vi "View-User Colors.vi"(11 "Material-Scheme.lvclass":refnum<class "Material-Scheme.lvclass">) -> ()   [LabVIEW 2021, in "TSC Material Theme.lvlib" / "Material-Scheme.lvclass"]
doc: "Allow developers to copy the colors from the scheme or save to the <i>User Colors</i> in the LabVIEW Configuration. \n\n<b>Note:</b> Updates to User Colors in the LabVIEW Config File require a restart\n\n<b>Code Developed By:</b>\nTechnology Service Corporation\nwww.tsc.com/atcs\n\nDeveloper:\nDaniel Coons"
uses:
  Material-Scheme.lvclass
  <vilib>/Utility/traverseref.llb/TRef TravTarget.ctl
  Material-Scheme.lvclass/Material-Scheme.ctl
  a595172c-2363-402c-a87e-7fcaa5b8fa44.vi
  <vilib>/Utility/colorconv.llb/Color to RGB.vi
  <vilib>/Comparison/Less/Less Functor/Less Functor.lvclass
  <vilib>/Utility/traverseref.llb/VI Scripting - Traverse.lvlib
panel:
  in  "exit":bool
  in  "stop VI":bool caption="This will FP Open to copy colors.\nUse Get Color tool or right click\nto copy color data."
  in  "restore LabVIEW defaults\nfor User Colors":bool
  in  "update User Colors":bool
  in  "deselect all":bool
  in  "default suggestions":bool
  out "selections":i32 caption="Numeric"
  in  "choices":bool[](array[boolean])
  out "color names":string[](array[string])
  out "Scrim":u32(colorbox)
  out "Shadow":u32(colorbox)
  out "Inverse Primary":u32(colorbox)
  out "Inverse on Surface":u32(colorbox)
  out "Inverse Surface":u32(colorbox)
  out "Outline Variant":u32(colorbox)
  out "Outline":u32(colorbox)
  out "On Surface Var":u32(colorbox)
  out "On Surface":u32(colorbox)
  out "Surf Container Highest":u32(colorbox)
  out "Surf Container High":u32(colorbox)
  out "Surf Container":u32(colorbox)
  out "Surf Container Low":u32(colorbox)
  out "Surf Container Lowest":u32(colorbox)
  out "Surface Bright":u32(colorbox)
  out "Surface":u32(colorbox)
  out "Surface Dim":u32(colorbox)
  out "On Error Container":u32(colorbox)
  out "Error Container":u32(colorbox)
  out "On Error":u32(colorbox)
  out "Error":u32(colorbox)
  out "On Tertiary Fixed Variant":u32(colorbox)
  out "On Tertiary Fixed":u32(colorbox)
  out "Tertiary Fixed Dim":u32(colorbox)
  out "Tertiary Fixed":u32(colorbox)
  out "On Tertiary Container":u32(colorbox)
  out "Tertiary Container":u32(colorbox)
  out "On Tertiary":u32(colorbox)
  out "Tertiary":u32(colorbox)
  out "On Secondary Fixed Variant":u32(colorbox)
  out "On Secondary Fixed":u32(colorbox)
  out "Secondary Fixed Dim":u32(colorbox)
  out "Secondary Fixed":u32(colorbox)
  out "On Secondary Container":u32(colorbox)
  out "Secondary Container":u32(colorbox)
  out "On Secondary":u32(colorbox)
  out "Secondary":u32(colorbox)
  out "On Primary Fixed Variant":u32(colorbox)
  out "On Primary Fixed":u32(colorbox)
  out "Primary Fixed Dim":u32(colorbox)
  out "Primary Fixed":u32(colorbox)
  out "On Primary Container":u32(colorbox)
  out "Primary Container":u32(colorbox)
  out "On Primary":u32(colorbox)
  out "Primary":u32(colorbox)
  out "hex colors":string[](array[string])
  # "developer can select\na maximum of 18 colors"
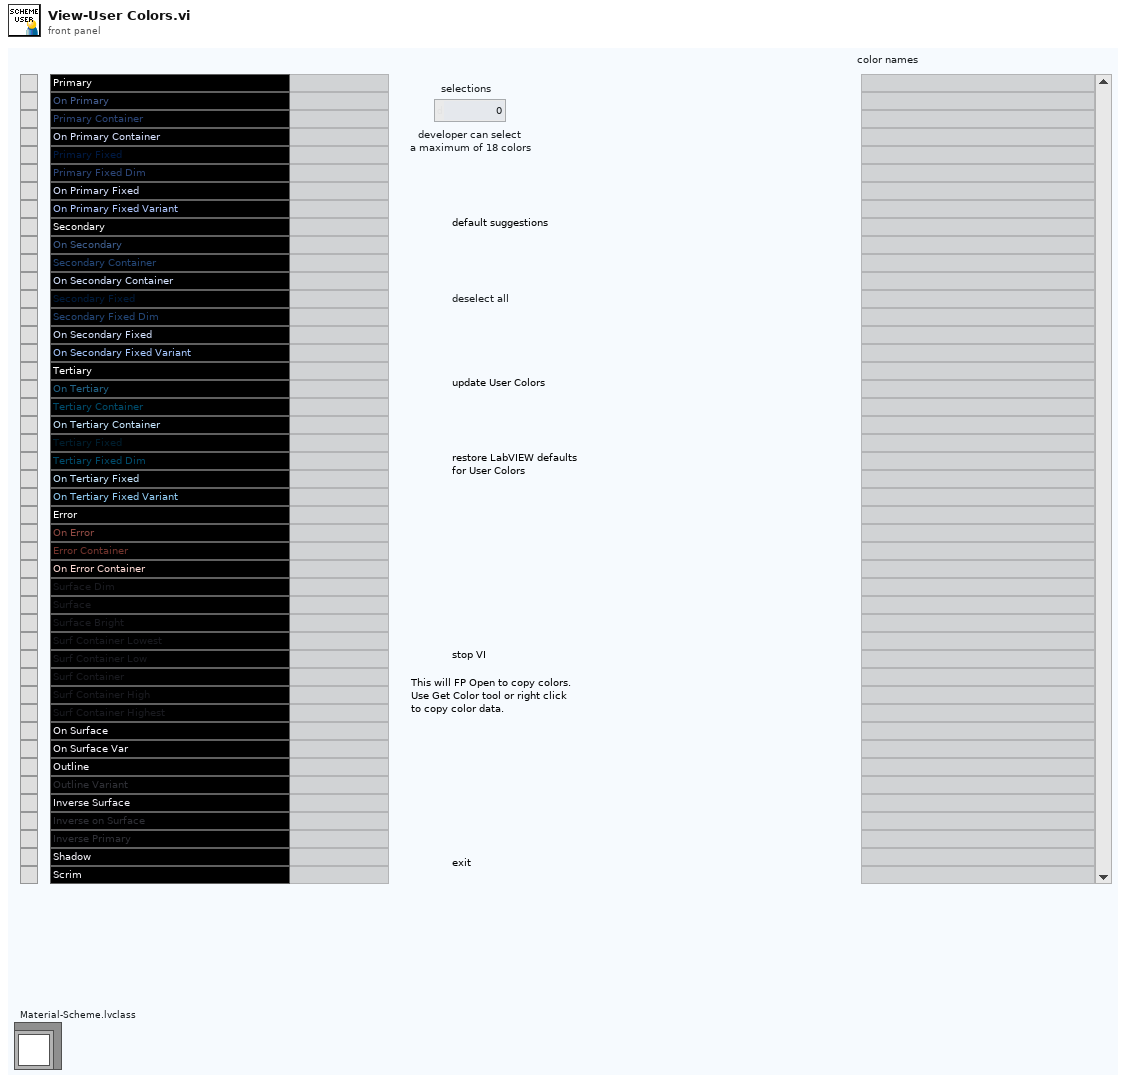
[diagram p1: front panel]
types:
  T1 = typedef "TRef TravTarget.ctl" = enum16{"FP", "BD", "Other"}
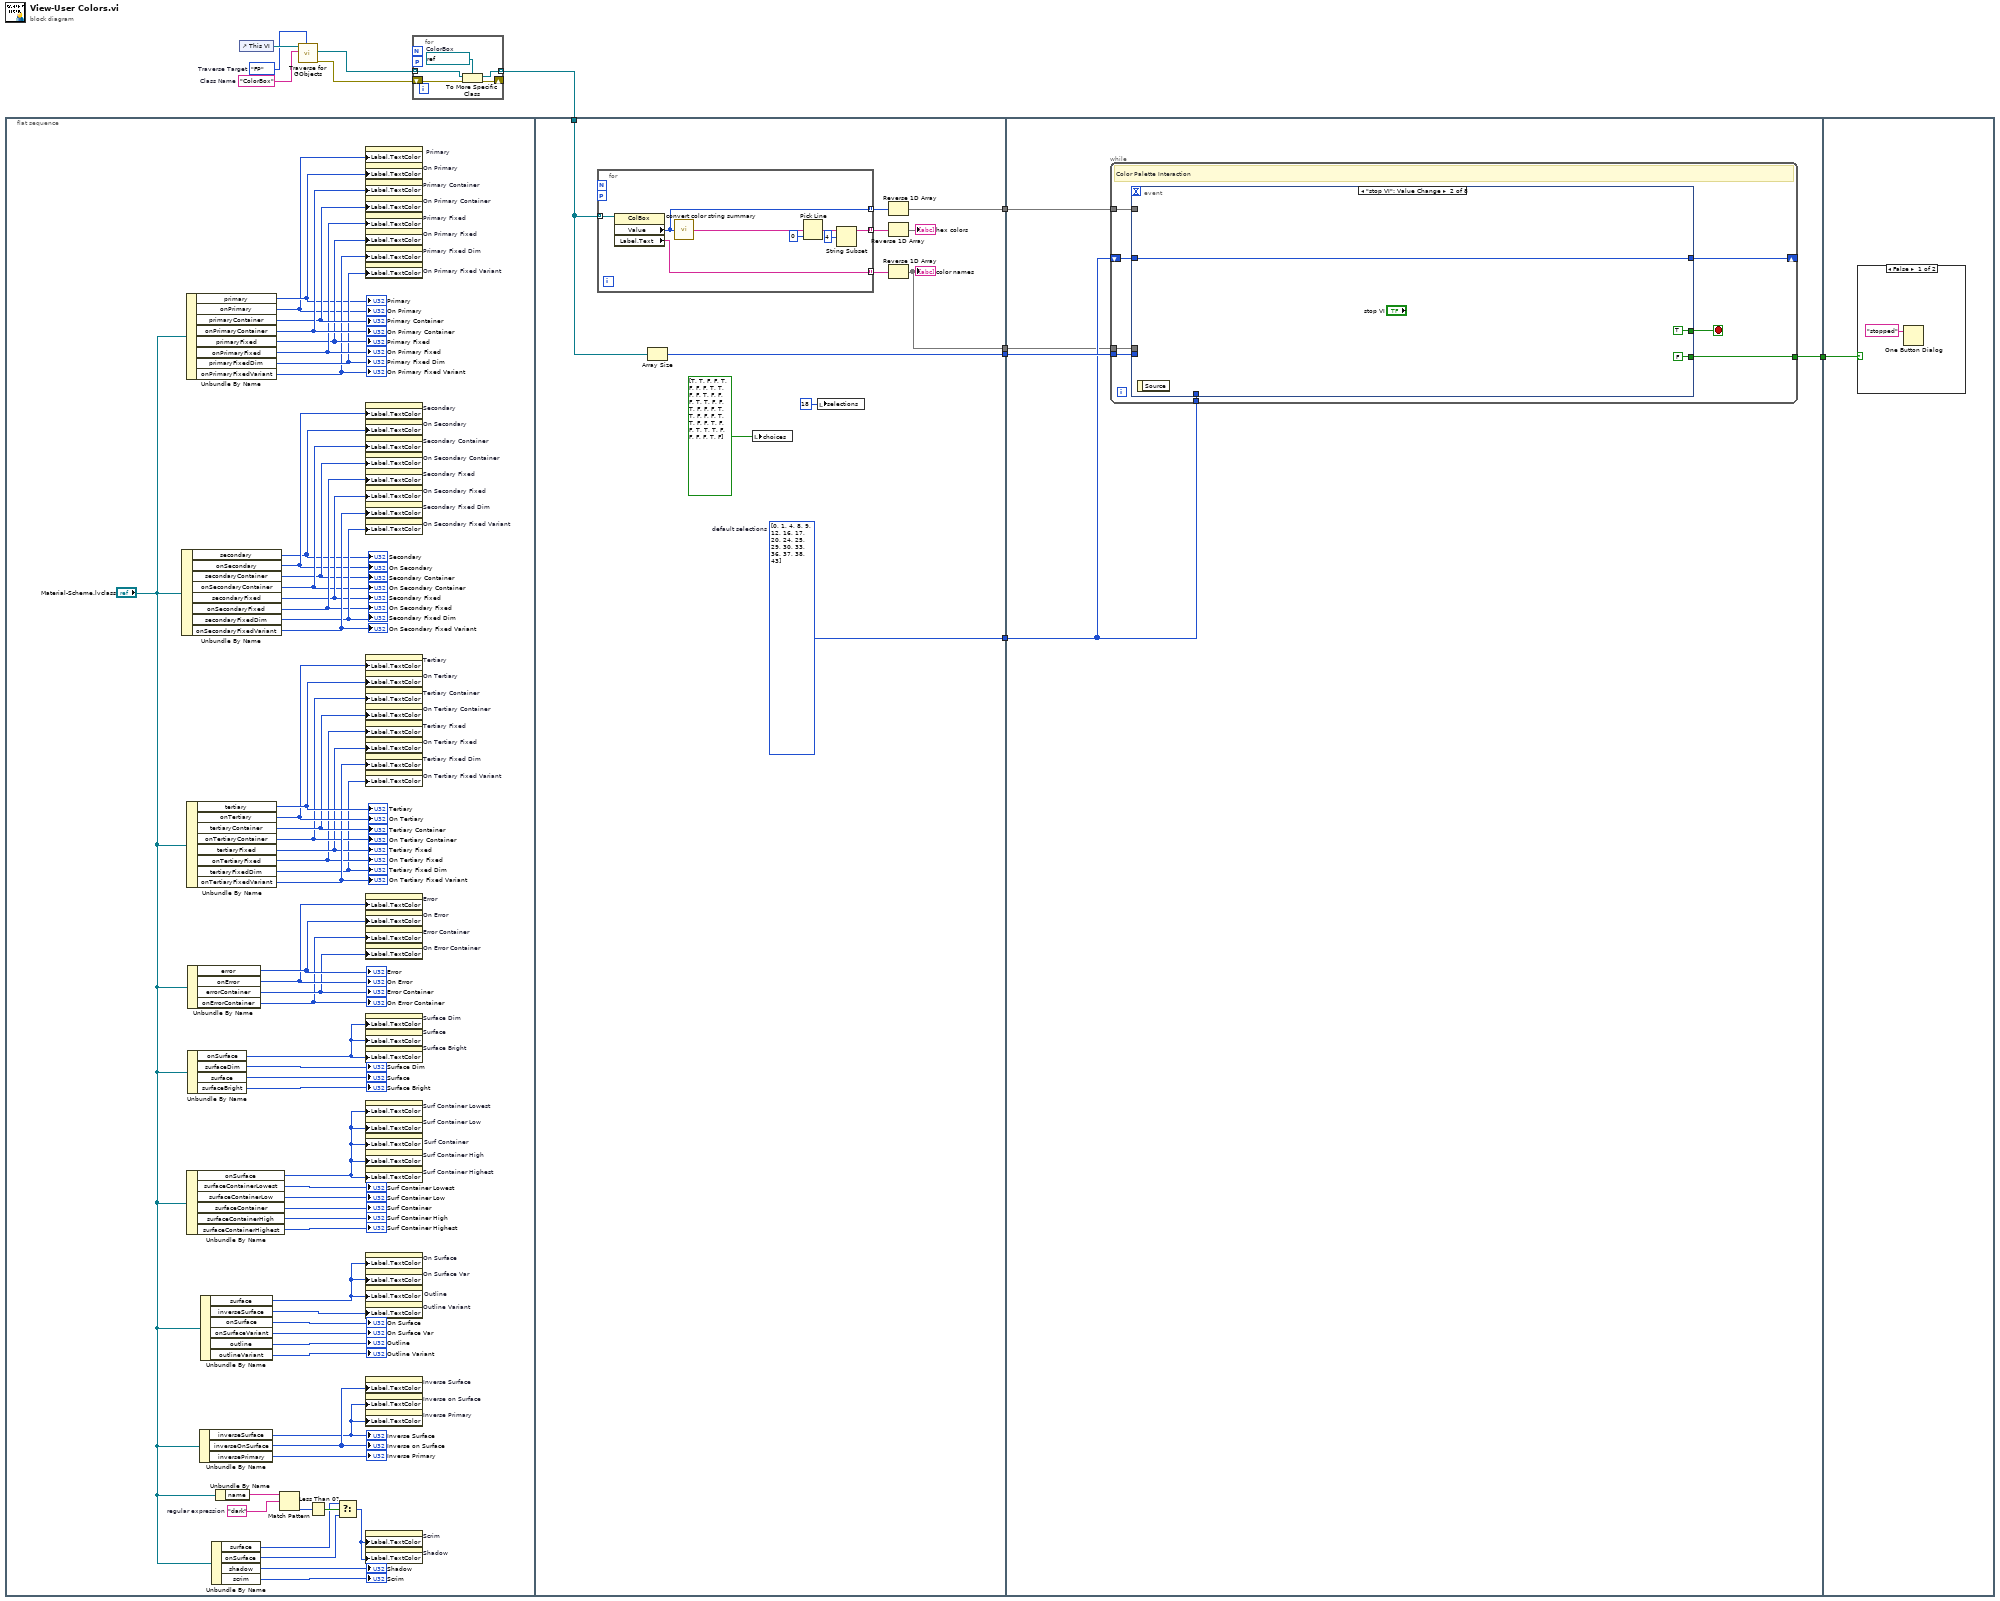
[diagram p0: block diagram]
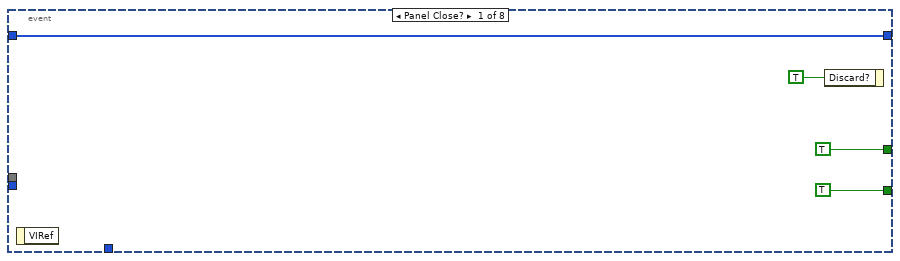
[diagram p2: hidden frame]
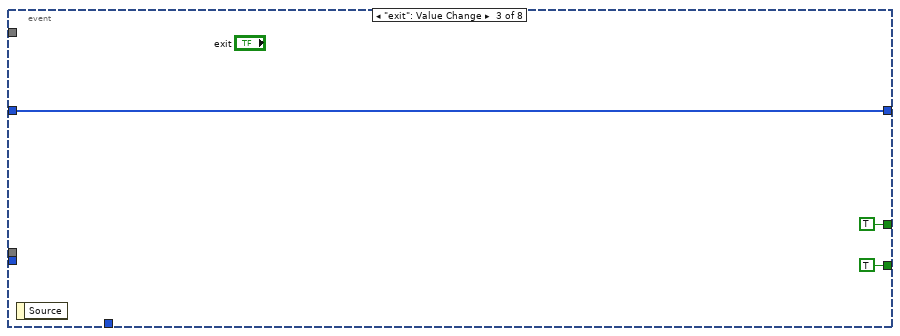
[diagram p3: hidden frame]
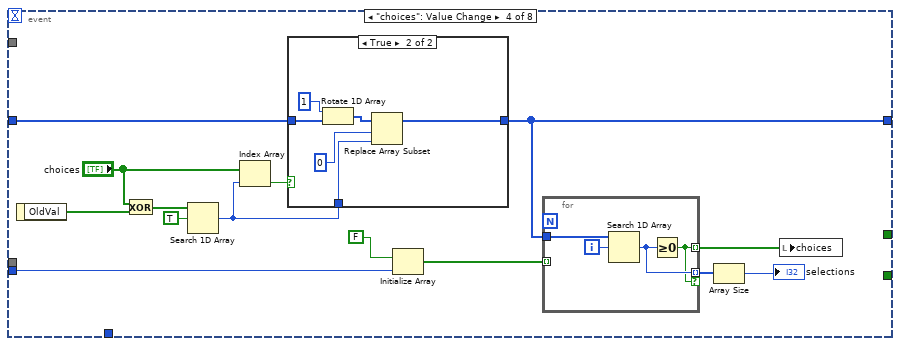
[diagram p4: hidden frame]
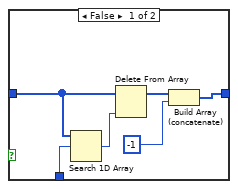
[diagram p5: hidden frame]
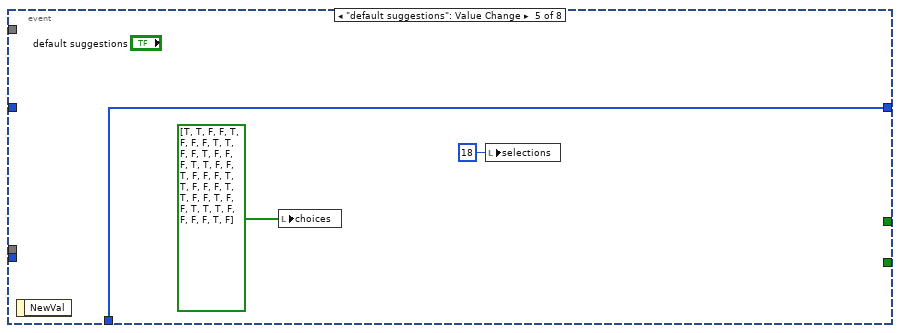
[diagram p6: hidden frame]
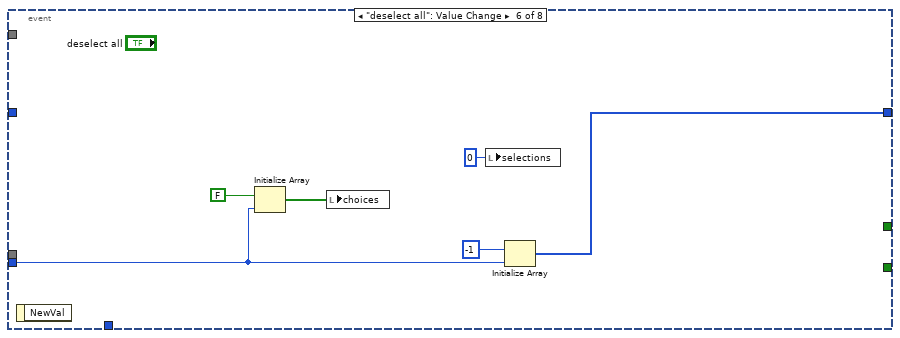
[diagram p7: hidden frame]
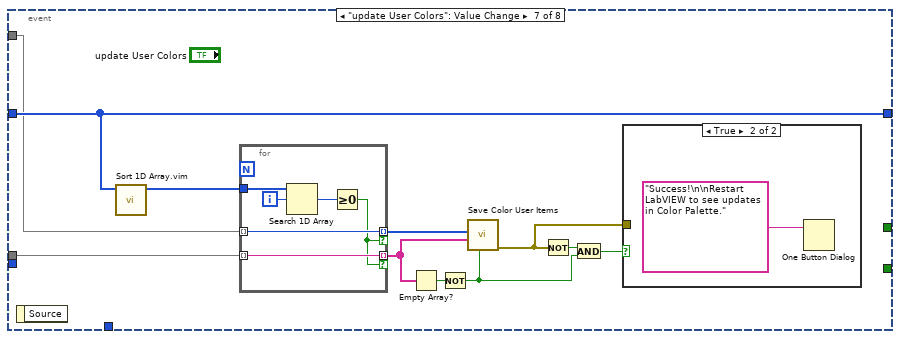
[diagram p8: hidden frame]
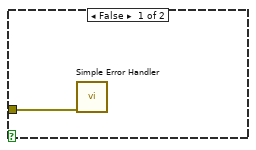
[diagram p9: hidden frame]
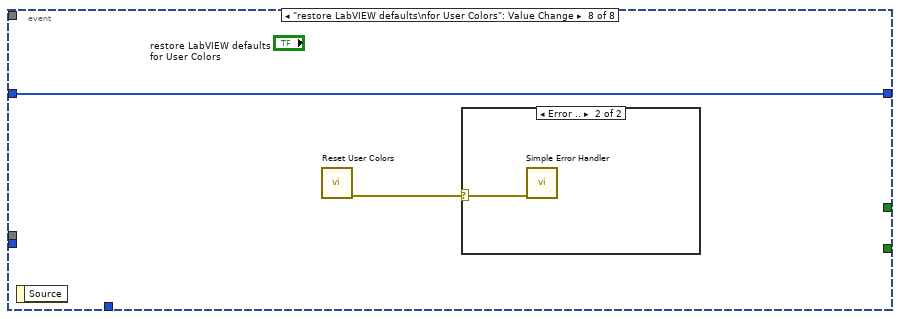
[diagram p10: hidden frame]
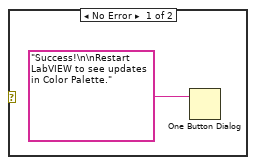
[diagram p11: hidden frame]
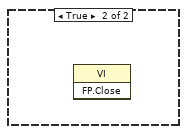
[diagram p12: hidden frame]
diagram:
  w8 = TRef_TravTarget."FP"  # Traverse Target
  w11 = "ColorBox"  # Class Name
  n1 = flat-sequence {
    tunnel: w6 -> [w76]
    tunnel: [w75] -> w5
    tunnel: [w72] -> w4
    tunnel: [w69] -> w3
    tunnel: [w70] -> w2
    tunnel: w5 -> [w92]
    tunnel: w4 -> [w91]
    tunnel: w3 -> [w90]
    tunnel: w2 -> [w89]
    tunnel: [w88] -> w1
    tunnel: w1 -> [w173]
    frame #0 {
      w19 = "dark"  # regular expression
      n2 = Unbundle By Name("Material-Scheme.lvclass") -> ("secondary"=w55:u32, "onSecondary"=w56:u32, "secondaryContainer"=w57:u32, "onSecondaryContainer"=w58:u32, "secondaryFixed"=w59:u32, "onSecondaryFixed"=w60:u32, "secondaryFixedDim"=w61:u32, "onSecondaryFixedVariant"=w62:u32)
      "Secondary" <- w55
      "On Secondary" <- w56
      "Secondary Container" <- w57
      "On Secondary Container" <- w58
      "Secondary Fixed Dim" <- w61
      "On Secondary Fixed" <- w60
      "On Secondary Fixed Variant" <- w62
      "Secondary Fixed" <- w59
      n3 = Unbundle By Name("Material-Scheme.lvclass") -> ("primary"=w13:u32, "onPrimary"=w12:u32, "primaryContainer"=w67:u32, "onPrimaryContainer"=w68:u32, "primaryFixed"=w65:u32, "onPrimaryFixed"=w66:u32, "primaryFixedDim"=w64:u32, "onPrimaryFixedVariant"=w63:u32)
      "Primary" <- w13
      "On Primary" <- w12
      "Primary Container" <- w67
      "On Primary Container" <- w68
      "Primary Fixed" <- w65
      "Primary Fixed Dim" <- w64
      "On Primary Fixed" <- w66
      "On Primary Fixed Variant" <- w63
      n4 = Unbundle By Name("Material-Scheme.lvclass") -> ("tertiary"=w54:u32, "onTertiary"=w53:u32, "tertiaryContainer"=w52:u32, "onTertiaryContainer"=w50:u32, "tertiaryFixed"=w49:u32, "onTertiaryFixed"=w48:u32, "tertiaryFixedDim"=w47:u32, "onTertiaryFixedVariant"=w51:u32)
      "Tertiary" <- w54
      "On Tertiary" <- w53
      "Tertiary Container" <- w52
      "On Tertiary Container" <- w50
      "Tertiary Fixed Dim" <- w47
      "On Tertiary Fixed" <- w48
      "On Tertiary Fixed Variant" <- w51
      "Tertiary Fixed" <- w49
      n5 = Unbundle By Name("Material-Scheme.lvclass") -> ("onSurface"=w33:u32, "surfaceContainerLowest"=→"Surf Container Lowest":u32, "surfaceContainerLow"=→"Surf Container Low":u32, "surfaceContainer"=→"Surf Container":u32, "surfaceContainerHigh"=→"Surf Container High":u32, "surfaceContainerHighest"=→"Surf Container Highest":u32)
      n6 = Unbundle By Name("Material-Scheme.lvclass") -> ("error"=w46:u32, "onError"=w45:u32, "errorContainer"=w44:u32, "onErrorContainer"=w43:u32)
      "Error" <- w46
      "On Error" <- w45
      "Error Container" <- w44
      "On Error Container" <- w43
      n7 = Unbundle By Name("Material-Scheme.lvclass") -> ("onSurface"=w39:u32, "surfaceDim"=→"Surface Dim":u32, "surface"=→"Surface":u32, "surfaceBright"=→"Surface Bright":u32)
      n8 = Unbundle By Name("Material-Scheme.lvclass") -> ("inverseSurface"=w24:u32, "inverseOnSurface"=w25:u32, "inversePrimary"=→"Inverse Primary":u32)
      "Inverse Surface" <- w24
      "Inverse on Surface" <- w25
      n9 = Unbundle By Name("Material-Scheme.lvclass") -> ("surface"=w28:u32, "inverseSurface"=w27:u32, "onSurface"=→"On Surface":u32, "onSurfaceVariant"=→"On Surface Var":u32, "outline"=→"Outline":u32, "outlineVariant"=→"Outline Variant":u32)
      n10 = Unbundle By Name("Material-Scheme.lvclass") -> ("surface"=w16:u32, "onSurface"=w15:u32, "shadow"=→"Shadow":u32, "scrim"=→"Scrim":u32)
      n11 = Unbundle By Name("Material-Scheme.lvclass") -> ("name"=w20:string)
      n12 = Match Pattern(string=w20, regular expression=w19) -> (offset past match=w18:i32)  [unwired: 1 in, 3 out]
      n13 = Less Than 0?(x=w18) -> (x < 0?=w17:bool)
      n14 = Select(t=w16, s=w17, f=w15) -> (s? t:f=w14:u32)
      n15 = property on="Primary" class="ColBox"("Label.TextColor"=w12) -> ()  [unwired: 2 in, 2 out]
      n16 = property on="On Primary" class="ColBox"("Label.TextColor"=w13) -> ()  [unwired: 2 in, 2 out]
      n17 = property on="Primary Container" class="ColBox"("Label.TextColor"=w68) -> ()  [unwired: 2 in, 2 out]
      n18 = property on="On Primary Container" class="ColBox"("Label.TextColor"=w67) -> ()  [unwired: 2 in, 2 out]
      n19 = property on="Primary Fixed" class="ColBox"("Label.TextColor"=w66) -> ()  [unwired: 2 in, 2 out]
      n20 = property on="On Primary Fixed" class="ColBox"("Label.TextColor"=w65) -> ()  [unwired: 2 in, 2 out]
      n21 = property on="Primary Fixed Dim" class="ColBox"("Label.TextColor"=w63) -> ()  [unwired: 2 in, 2 out]
      n22 = property on="On Primary Fixed Variant" class="ColBox"("Label.TextColor"=w64) -> ()  [unwired: 2 in, 2 out]
      n23 = property on="Secondary" class="ColBox"("Label.TextColor"=w56) -> ()  [unwired: 2 in, 2 out]
      n24 = property on="On Secondary" class="ColBox"("Label.TextColor"=w55) -> ()  [unwired: 2 in, 2 out]
      n25 = property on="Secondary Container" class="ColBox"("Label.TextColor"=w58) -> ()  [unwired: 2 in, 2 out]
      n26 = property on="On Secondary Container" class="ColBox"("Label.TextColor"=w57) -> ()  [unwired: 2 in, 2 out]
      n27 = property on="Secondary Fixed" class="ColBox"("Label.TextColor"=w60) -> ()  [unwired: 2 in, 2 out]
      n28 = property on="On Secondary Fixed" class="ColBox"("Label.TextColor"=w59) -> ()  [unwired: 2 in, 2 out]
      n29 = property on="Secondary Fixed Dim" class="ColBox"("Label.TextColor"=w62) -> ()  [unwired: 2 in, 2 out]
      n30 = property on="On Secondary Fixed Variant" class="ColBox"("Label.TextColor"=w61) -> ()  [unwired: 2 in, 2 out]
      n31 = property on="Tertiary" class="ColBox"("Label.TextColor"=w53) -> ()  [unwired: 2 in, 2 out]
      n32 = property on="On Tertiary" class="ColBox"("Label.TextColor"=w54) -> ()  [unwired: 2 in, 2 out]
      n33 = property on="Tertiary Container" class="ColBox"("Label.TextColor"=w50) -> ()  [unwired: 2 in, 2 out]
      n34 = property on="On Tertiary Container" class="ColBox"("Label.TextColor"=w52) -> ()  [unwired: 2 in, 2 out]
      n35 = property on="Tertiary Fixed" class="ColBox"("Label.TextColor"=w48) -> ()  [unwired: 2 in, 2 out]
      n36 = property on="On Tertiary Fixed" class="ColBox"("Label.TextColor"=w49) -> ()  [unwired: 2 in, 2 out]
      n37 = property on="Tertiary Fixed Dim" class="ColBox"("Label.TextColor"=w51) -> ()  [unwired: 2 in, 2 out]
      n38 = property on="On Tertiary Fixed Variant" class="ColBox"("Label.TextColor"=w47) -> ()  [unwired: 2 in, 2 out]
      n39 = property on="Error" class="ColBox"("Label.TextColor"=w45) -> ()  [unwired: 2 in, 2 out]
      n40 = property on="On Error" class="ColBox"("Label.TextColor"=w46) -> ()  [unwired: 2 in, 2 out]
      n41 = property on="Error Container" class="ColBox"("Label.TextColor"=w43) -> ()  [unwired: 2 in, 2 out]
      n42 = property on="On Error Container" class="ColBox"("Label.TextColor"=w44) -> ()  [unwired: 2 in, 2 out]
      n43 = property on="Surface Dim" class="ColBox"("Label.TextColor"=w39) -> ()  [unwired: 2 in, 2 out]
      n44 = property on="Surface" class="ColBox"("Label.TextColor"=w39) -> ()  [unwired: 2 in, 2 out]
      n45 = property on="Surface Bright" class="ColBox"("Label.TextColor"=w39) -> ()  [unwired: 2 in, 2 out]
      n46 = property on="Surf Container Lowest" class="ColBox"("Label.TextColor"=w33) -> ()  [unwired: 2 in, 2 out]
      n47 = property on="Surf Container Low" class="ColBox"("Label.TextColor"=w33) -> ()  [unwired: 2 in, 2 out]
      n48 = property on="Surf Container" class="ColBox"("Label.TextColor"=w33) -> ()  [unwired: 2 in, 2 out]
      n49 = property on="Surf Container High" class="ColBox"("Label.TextColor"=w33) -> ()  [unwired: 2 in, 2 out]
      n50 = property on="Surf Container Highest" class="ColBox"("Label.TextColor"=w33) -> ()  [unwired: 2 in, 2 out]
      n51 = property on="On Surface" class="ColBox"("Label.TextColor"=w28) -> ()  [unwired: 2 in, 2 out]
      n52 = property on="On Surface Var" class="ColBox"("Label.TextColor"=w28) -> ()  [unwired: 2 in, 2 out]
      n53 = property on="Outline" class="ColBox"("Label.TextColor"=w28) -> ()  [unwired: 2 in, 2 out]
      n54 = property on="Outline Variant" class="ColBox"("Label.TextColor"=w27) -> ()  [unwired: 2 in, 2 out]
      n55 = property on="Inverse Surface" class="ColBox"("Label.TextColor"=w25) -> ()  [unwired: 2 in, 2 out]
      n56 = property on="Inverse on Surface" class="ColBox"("Label.TextColor"=w24) -> ()  [unwired: 2 in, 2 out]
      n57 = property on="Inverse Primary" class="ColBox"("Label.TextColor"=w24) -> ()  [unwired: 2 in, 2 out]
      n58 = property on="Scrim" class="ColBox"("Label.TextColor"=w14) -> ()  [unwired: 2 in, 2 out]
      n59 = property on="Shadow" class="ColBox"("Label.TextColor"=w14) -> ()  [unwired: 2 in, 2 out]
    }
    frame #1 {
      w72 = i32[] [0, 1, 4, 8, 9, 12, 16, 17, 20, 24, 25, 29, 30, 33, 36, 37, 38, 43]  # default selections
      n60 = for {
        tunnel: w76 -> [w87] mode=indexing
        workers-P: _ -> [_]
        tunnel: [w82] -> w79 mode=indexing
        tunnel: [w83] -> w78 mode=indexing
        tunnel: [w80] -> w71 mode=indexing
        n61 = property class="ColBox"(reference=w87) -> ("Value"=w80:u32, "Label.Text"=w83:string)  [unwired: 1 in, 2 out]
        n62 = call "convert color string summary.vi"("primary"=w80) -> ("String"=w86:string)
        n63 = Pick Line(multi-line string=w86, line index=0) -> (output string=w85:string)  [unwired: 1 in]
        n64 = String Subset(string=w85, offset (0)=4) -> (substring=w82:string)  [unwired: 1 in]
      }
      n65 = Array Size(array=w76) -> (size(s)=w75:i32)
      n66 = local write "choices"(bool[] [TRUE, TRUE, FALSE, FALSE, TRUE, FALSE, FALSE, FALSE, TRUE, TRUE, FALSE, FALSE, TRUE, FALSE, FALSE, FALSE, TRUE, TRUE, FALSE, FALSE, TRUE, FALSE, FALSE, FALSE, TRUE, TRUE, FALSE, FALSE, FALSE, TRUE, TRUE, FALSE, FALSE, TRUE, FALSE, FALSE, TRUE, TRUE, TRUE, FALSE, FALSE, FALSE, FALSE, TRUE, FALSE] ("choices")) -> ()
      n67 = local write "selections"(18 ("selections")) -> ()
      n68 = Reverse 1D Array(array=w71) -> (reversed array=w69:u32[])
      n69 = Reverse 1D Array(array=w79) -> (reversed array=→"hex colors":string[])
      n70 = Reverse 1D Array(array=w78) -> (reversed array=w70:string[])
      "color names" <- w70
    }
    frame #2 {
      n71 = while {
        shift-right: [w98] -> _
        shift-left: w91 -> [w99]
        tunnel: w92 -> [w97]
        tunnel: w91 -> [w96]
        tunnel: w90 -> [w95]
        tunnel: w89 -> [w94]
        tunnel: [w93] -> w88
        stop <- w100 stop-if-true
        # "Color Palette Interaction"
        n72 = event shown="[1] \"stop VI\": Value Change" {
          selector: _ -> [_ _ _ _ _ _ _ _]
          dyn-events: _ -> [_ _ _ _ _ _ _ _]
          timeout: _ -> [_ _ _ _ _ _ _ _]
          tunnel: [TRUE TRUE TRUE _ _ _ _ _] -> w100
          tunnel: w99 -> [w102 w107 w110 w124 _ _ w160 w170]
          tunnel: [w102 w107 w110 w113 w143 w144 w160 w170] -> w98
          tunnel: w97 -> [_ _ _ w116 _ w145 _ _]
          tunnel: w96 -> [_ _ _ _ w143 _ _ _]
          tunnel: w95 -> [_ _ _ _ _ _ w158 _]
          tunnel: w94 -> [_ _ _ _ _ _ w157 _]
          tunnel: [TRUE FALSE TRUE _ _ _ _ _] -> w93
          event Panel Close? {
            n73 = event-data() -> ()  [unwired: 1 in, 1 out]
            n74 = event-data("Discard?"=TRUE) -> ()  [unwired: 1 in, 1 out]
          }
          event "stop VI": Value Change {
            n75 = event-data() -> ()  [unwired: 1 in, 1 out]
          }
          event "exit": Value Change {
            n76 = event-data() -> ()  [unwired: 1 in, 1 out]
          }
          event "choices": Value Change {
            n77 = event-data() -> ("OldVal"=w123:bool[])  [unwired: 1 in]
            n78 = Exclusive Or(1:w123, 2:"choices") -> (0:w122:bool[])
            n79 = Search 1D Array(1D array=w122, element=TRUE) -> (index of element=w119:i32)  [unwired: 1 in]
            n80 = Index Array(array="choices", index=w119) -> (element=w118:bool)
            n81 = case shown="True" w118 {
              tunnel: w124 -> [w133 w138]
              tunnel: [w130 w136] -> w113
              tunnel: w119 -> [w132 w140]
              frame False {
                n82 = Search 1D Array(1D array=w133, element=w132) -> (index of element=w131:i32)  [unwired: 1 in]
                n83 = Delete From Array(array=w133, index=w131) -> (array with subset deleted=w134:i32[])  [unwired: 1 in, 1 out]
                n84 = Build Array (concatenate)(w134, -1 ("element")) -> (w130:i32[])
              }
              frame True {
                n85 = Rotate 1D Array(1:w138, 2:1 ("n")) -> (0:w137:i32[])
                n86 = Replace Array Subset(array=w137, new element=w140, index=0) -> (w136:i32[])
              }
            }
            n87 = Initialize Array(FALSE, w116) -> (w115:bool[])
            n88 = for {
              tunnel: w115 -> [_] mode=indexing
              tunnel: w113 -> [w128]
              tunnel: [w125] -> w114 mode=indexing
              tunnel: [w126] -> w112 mode=indexing if=w125
              i -> [w127]
              n89 = Search 1D Array(1D array=w128, element=w127) -> (index of element=w126:i32)  [unwired: 1 in]
              n90 = Greater Or Equal To 0?(x=w126) -> (x >= 0?=w125:bool)
            }
            n91 = Array Size(array=w112) -> (size(s)=→"selections":i32)
            n92 = local write "choices"(w114) -> ()
          }
          event "default suggestions": Value Change {
            n93 = event-data() -> ()  [unwired: 1 in, 1 out]
            n94 = local write "choices"(bool[] [TRUE, TRUE, FALSE, FALSE, TRUE, FALSE, FALSE, FALSE, TRUE, TRUE, FALSE, FALSE, TRUE, FALSE, FALSE, FALSE, TRUE, TRUE, FALSE, FALSE, TRUE, FALSE, FALSE, FALSE, TRUE, TRUE, FALSE, FALSE, FALSE, TRUE, TRUE, FALSE, FALSE, TRUE, FALSE, FALSE, TRUE, TRUE, TRUE, FALSE, FALSE, FALSE, FALSE, TRUE, FALSE] ("choices")) -> ()
            n95 = local write "selections"(18 ("selections")) -> ()
          }
          event "deselect all": Value Change {
            n96 = event-data() -> ()  [unwired: 1 in, 1 out]
            n97 = Initialize Array(FALSE, w145) -> (w147:bool[])
            n98 = local write "choices"(w147) -> ()
            n99 = local write "selections"(0 ("selections")) -> ()
            n100 = Initialize Array(-1, w145) -> (w144:i32[])
          }
          event "update User Colors": Value Change {
            n101 = event-data() -> ()  [unwired: 1 in, 1 out]
            n102 = call "Sort 1D Array.vim"("unsorted array"=w160) -> ("sorted array"=w159:i32[])  [unwired: 10 in]
            n103 = for {
              tunnel: w159 -> [w168]
              tunnel: w158 -> [w165] mode=indexing
              tunnel: [w165] -> w156 mode=indexing if=w163
              tunnel: w157 -> [w164] mode=indexing
              tunnel: [w164] -> w155 mode=indexing if=w163
              i -> [w167]
              n104 = Search 1D Array(1D array=w168, element=w167) -> (index of element=w166:i32)  [unwired: 1 in]
              n105 = Greater Or Equal To 0?(x=w166) -> (x >= 0?=w163:bool)
            }
            n106 = Empty Array?(array=w155) -> (empty?=w154:bool)
            n107 = Not(x=w154) -> (.not. x?=w153:bool)
            n108 = call "Save Color User Items.vi"("save settings?"=w153, "Color Names"=w155, "colors"=w156) -> ("error out"=w150:errorcluster)  [unwired: 8 in]
            n109 = Not(x=w150) -> (.not. x?=w152:bool)
            n110 = And(x=w152, y=w153) -> (x .and. y?=w151:bool)
            n111 = case shown="True" w151 {
              tunnel: w150 -> [w161 _]
              frame False {
                n112 = call <vilib>:"Simple Error Handler.vi"("error in (no error)"=w161) -> ()  [unwired: 4 in, 5 out]
              }
              frame True {
                n113 = One Button Dialog(message="Success!\n\nRestart LabVIEW to see updates in Color Palette.") -> ()  [unwired: 1 in, 1 out]
              }
            }
          }
          event "restore LabVIEW defaults\nfor User Colors": Value Change {
            n114 = event-data() -> ()  [unwired: 1 in, 1 out]
            n115 = call "Reset User Colors.vi"() -> ("error out"=w169:errorcluster)  [unwired: 11 in]
            n116 = case shown="Error .." w169 {
              selector: w169 -> [_ w172]
              frame No Error {
                n117 = One Button Dialog(message="Success!\n\nRestart LabVIEW to see updates in Color Palette.") -> ()  [unwired: 1 in, 1 out]
              }
              frame Error {
                n118 = call <vilib>:"Simple Error Handler.vi"("error in (no error)"=w172) -> ()  [unwired: 4 in, 5 out]
              }
            }
          }
        }
      }
    }
    frame #3 {
      n119 = case shown="False" w173 {
        frame False {
          n120 = One Button Dialog(message="stopped") -> ()  [unwired: 1 in, 1 out]
        }
        frame True {
          n121 = invoke class="VI" method="FP.Close"() -> ()  [unwired: 3 in, 3 out]
        }
      }
    }
  }
  n122 = control-ref of="This VI"() -> (w10:refnum<vi>)
  n123 = call <vilib>:"Traverse for GObjects.vi"("Traverse Target"=w8, "Class Name"=w11, "VI Refnum"=w10) -> ("error out"=w7:errorcluster, "References"=w9:refnum<vi>[])  [unwired: 5 in, 2 out]
  n124 = for {
    tunnel: w9 -> [w176] mode=indexing
    shift-right: [w178] -> _
    shift-left: w7 -> [w179]
    tunnel: [w175] -> w6 mode=indexing
    workers-P: _ -> [_]
    w177 = refnum<vi> refnum  # ColorBox
    n125 = To More Specific Class(target class=w177, reference=w176, error in=w179) -> (specific class reference=w175:refnum<vi>, error out=w178:errorcluster)
  }
